vi "Force Rename Item.vi"(8 "error in":errorcluster, 10 "String":string, 11 "Item Ref":T1 format="%.0x") -> (0 "error out":errorcluster, 3 "Item Ref out":T1 format="%.0x")   [LabVIEW 2011, in "AIT 1553 Custom Device.lvlib"]
uses:
  AIT 1553 Custom Device.lvlib
  <vilib>/NI Veristand/Custom Device API/Custom Device Item Ref.ctl
  NationalInstruments.VeriStand.SystemStorage
  <vilib>/NI Veristand/Custom Device API/Custom Device API.lvlib
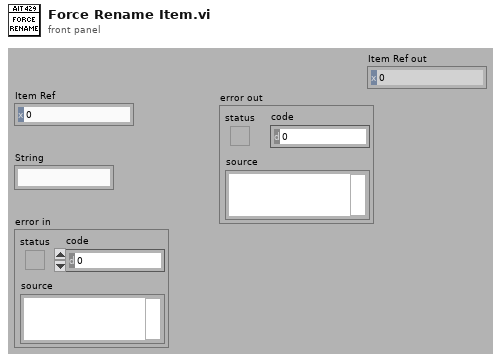
[diagram p1: front panel]
types:
  T1 = typedef "Custom Device API.lvlib/Custom Device Item Ref.ctl" = u64
  T2 = typedef "Custom Device API.lvlib/Custom Device Pointer.ctl" = refnum<k24>
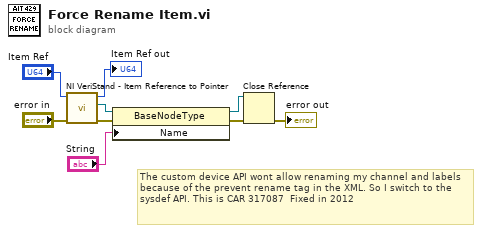
[diagram p0: block diagram]
diagram:
  # "The custom device API wont allow renaming my channel and labels because of the prevent rename tag in the XML. So I switch to the sysdef API. This is CAR 317087  Fixed in 2012"
  n1 = call <vilib>:"NI VeriStand - Item Reference to Pointer.vi"("error in (no error)"="error in", "Item Ref in"="Item Ref") -> ("error out"=w6:errorcluster, "Node Pointer"=w7:T2, "Item Ref out"=→"Item Ref out":T1)  [unwired: 6 in, 1 out]
  n2 = property class="BaseNodeType"(reference=w7, error in=w6, "Name"="String") -> (reference out=w3:T2, error out=w4:errorcluster)
  n3 = Close Reference(reference=w3, error in (no error)=w4) -> (error out=→"error out":errorcluster)
